vi "FL_DEC_split_and_filter.vi"(4 "Filter type":u16(ring)=5 items=["None", "Kalman 0.50", "Kalman 0.30", "Kalman 0.12", "Savitzky-Golay 3/5", "Savitzky-Golay 3/11", "Savitzky-Golay 3/31", ""], 5 "InputArray":sgl[](array[numeric])) -> (1 "Output cluster":cluster{"X1":dbl, "Y1":dbl, "X2":dbl, "Y2":dbl})   [LabVIEW 2018]
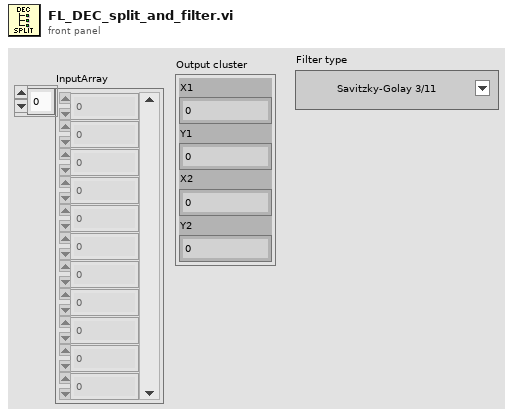
[diagram p1: front panel]
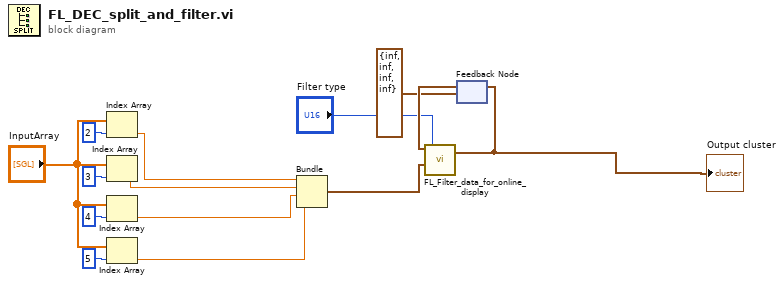
[diagram p0: block diagram]
diagram:
  n1 = Index Array(array="InputArray", index=2 ("disabled index (col)")) -> (element=w9:sgl)
  n2 = Index Array(array="InputArray", index=3 ("disabled index (col)")) -> (element=w8:sgl)
  n3 = Index Array(array="InputArray", index=4 ("disabled index (col)")) -> (element=w7:sgl)
  n4 = Index Array(array="InputArray", index=5 ("disabled index (col)")) -> (element=w6:sgl)
  n5 = Bundle(w9, w8, w7, w6) -> (w5:cluster{sgl, sgl, sgl, sgl})  [unwired: 1 in]
  n6 = feedback #1(cluster{"X1":dbl, "Y1":dbl, "X2":dbl, "Y2":dbl} {"X1"=inf, "Y1"=inf, "X2"=inf, "Y2"=inf} ("Output data")) -> (w4:cluster{"X1":dbl, "Y1":dbl, "X2":dbl, "Y2":dbl})
  n7 = call "FL_Filter_data_for_online_display.vi"("Input data"=w5, "Filter type"="Filter type", "Data filtered on previous step"=w4) -> ("Output data"=w1:cluster{"X1":dbl, "Y1":dbl, "X2":dbl, "Y2":dbl})  [unwired: 2 in]
  "Output cluster" <- w1
  n8 = feedback-in #1(w1) -> ()
